vi "Report Calculate Data.vi"(7 "Channels #":i32, 8 "error in (no error)":errorcluster, 9 "Report SP":i32[](array[numeric]), 10 "Group Names":string[](array[string]), 11 "Refnum in":refnum<k34>) -> (0 "error out":errorcluster, 1 "Max Array Report":i32[][](array[numeric]), 2 "Mean Array Report":i32[][](array[numeric]), 3 "Refnum out":refnum<k34>, 4 "Mean Array":i32[][](array[numeric]), 5 "ALL Points":i32[](array[numeric]), 6 "Max Array":i32[][](array[numeric]))   [LabVIEW 2020]
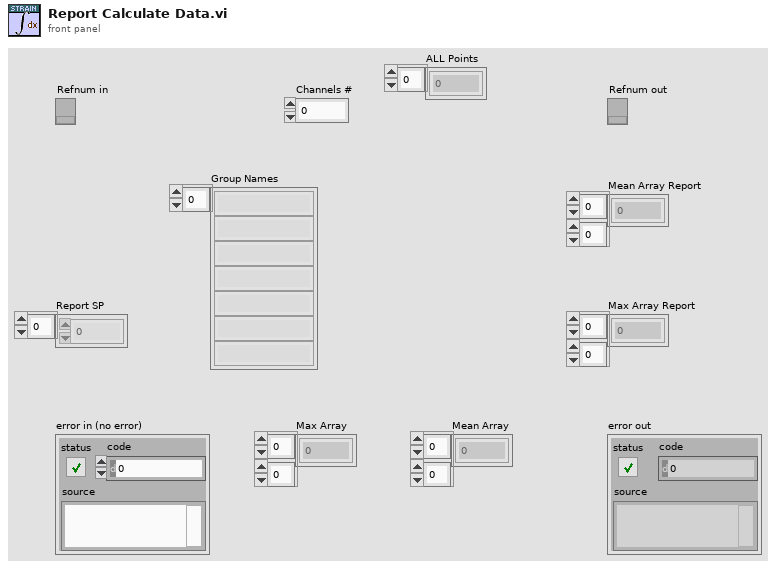
[diagram p1: front panel]
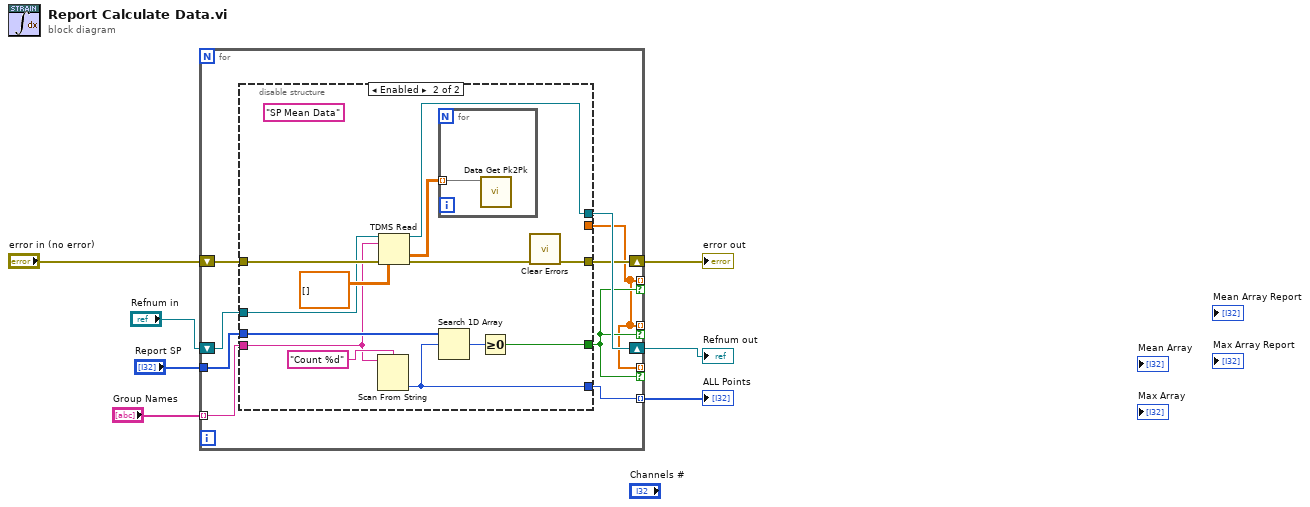
[diagram p0: block diagram]
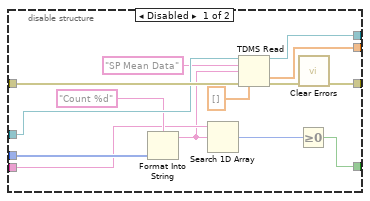
[diagram p2: hidden frame]
diagram:
  n1 = for {
    tunnel: [w8] -> _ mode=indexing if=w10
    shift-right: [w11] -> w4
    shift-left: "error in (no error)" -> [w15]
    shift-right: [w16] -> w2
    shift-left: "Refnum in" -> [w14]
    tunnel: "Report SP" -> [w13]
    tunnel: "Group Names" -> [w12] mode=indexing
    tunnel: [w8] -> _ mode=indexing if=w10
    tunnel: [w8] -> _ mode=indexing if=w10
    tunnel: [w9] -> w3 mode=indexing
    n2 = disable-structure shown="Enabled" {
      disable-tunnel: [w30 w43] -> w16
      disable-tunnel: w15 -> [w27 w40]
      disable-tunnel: w14 -> [w26 w39]
      disable-tunnel: [w25 _] -> w8
      disable-tunnel: w13 -> [w23 w33]
      disable-tunnel: [w21 w38] -> w10
      disable-tunnel: w12 -> [w20 w31]
      disable-tunnel: [w17 w36] -> w11
      disable-tunnel: [_ w32] -> w9
      frame Disabled {
        n3 = Format Into String(format string="Count %d" ("group name in (Untitled)"), w23) -> (resulting string=w19:string)  [unwired: 2 in, 1 out]
        n4 = Search 1D Array(1D array=w20, element=w19) -> (index of element=w18:i32)  [unwired: 1 in]
        n5 = TDMS Read(0:w26, 5:"SP Mean Data" ("group name in"), 7:w19, 11:w27, 12:dbl[] []) -> (4:w30:refnum<k34>, 10:w25:dbl[], 15:w28:errorcluster)  [unwired: 3 in, 3 out]
        n6 = Greater Or Equal To 0?(x=w18) -> (x >= 0?=w21:bool)
        n7 = call <vilib>:"Clear Errors.vi"("error in (no error)"=w28) -> ("error out"=w17:errorcluster)  [unwired: 5 in, 1 out]
      }
      frame Enabled {
        (unwired) "SP Mean Data" ("group name in")
        n8 = Scan From String(format string="Count %d", input string=w31) -> (output 1=w32:i32)  [unwired: 3 in, 3 out]
        n9 = TDMS Read(0:w39, 5:w31, 11:w40, 12:dbl[][] []) -> (4:w43:refnum<k34>, 10:w35:dbl[][], 15:w41:errorcluster)  [unwired: 4 in, 3 out]
        n10 = for {
          tunnel: w35 -> [w44] mode=indexing
          n11 = call "Data Get Pk2Pk.vi"("Data"=w44) -> ()  [unwired: 10 in, 1 out]
        }
        n12 = Search 1D Array(1D array=w33, element=w32) -> (index of element=w37:i32)  [unwired: 1 in]
        n13 = Greater Or Equal To 0?(x=w37) -> (x >= 0?=w38:bool)
        n14 = call <vilib>:"Clear Errors.vi"("error in (no error)"=w41) -> ("error out"=w36:errorcluster)  [unwired: 5 in, 1 out]
      }
    }
  }
  "error out" <- w4
  "Refnum out" <- w2
  "ALL Points" <- w3
